vi "WMI Shutdown.vi"() -> ()   [LabVIEW 2012]
uses:
  System.Management
panel:
  out "error out":errorcluster
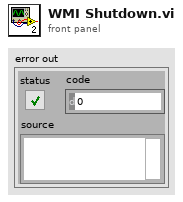
[diagram p1: front panel]
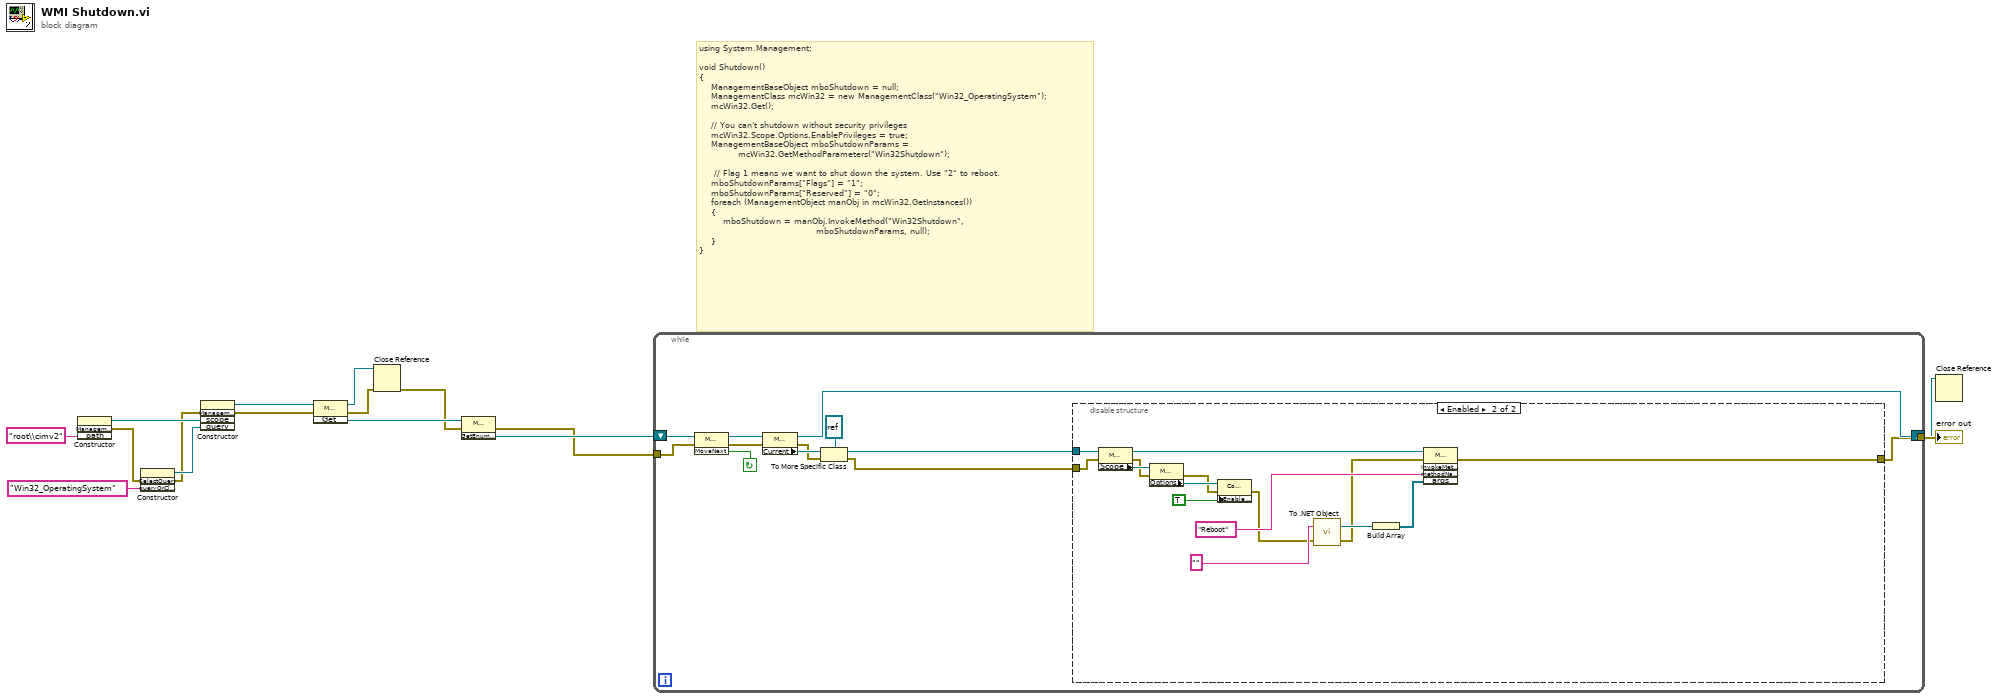
[diagram p0: block diagram]
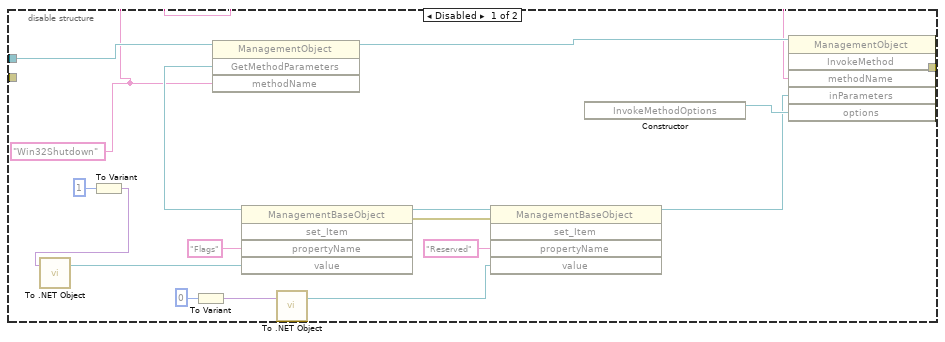
[diagram p2: hidden frame]
diagram:
  # "using System.Management;\n\nvoid Shutdown()\n{\n    ManagementBaseObject mboShutdown = null;\n    ManagementClass mcWin32 = new ManagementClass(\"Win32_OperatingSystem\");\n    mcWin32.Get();\n\n    // You can't shutdown without security privileges\n    mcWin32.Scope.Options.EnablePrivileges = true;\n    ManagementBaseObject mboShutdownParams =\n             mcWin32.GetMethodParameters(\"Win32Shutdown\");\n\n     // Flag 1 means we want to shut down the system. Use \"2\" to reboot.\n    mboShutdownParams[\"Flags\"] = \"1\";\n    mboShutdownParams[\"Reserved\"] = \"0\";\n    foreach (ManagementObject manObj in mcWin32.GetInstances())\n    {\n        mboShutdown = manObj.InvokeMethod(\"Win32Shutdown\", \n                                       mboShutdownParams, null);\n    }\n}"
  n1 = constructor class="ManagementScope"("path"="root\\cimv2" ("Scope")) -> (reference out=w14:refnum<k24>, error out=w2:errorcluster)  [unwired: 3 in, 2 out]
  n2 = constructor class="SelectQuery"(error in=w2, "queryOrClassName"="Win32_OperatingSystem") -> (reference out=w13:refnum<k24>, error out=w1:errorcluster)  [unwired: 2 in, 2 out]
  n3 = constructor class="ManagementObjectSearcher"(error in=w1, "scope"=w14, "query"=w13) -> (reference out=w3:refnum<k24>, error out=w10:errorcluster)  [unwired: 2 in, 3 out]
  n4 = invoke class="ManagementObjectSearcher" method="Get"(reference=w3, error in=w10) -> (reference out=w7:refnum<k24>, error out=w6:errorcluster, "Get"=w12:refnum<k24>)  [unwired: 1 in]
  n5 = Close Reference(reference=w7, error in (no error)=w6) -> (error out=w5:errorcluster)
  n6 = invoke class="ManagementObjectCollection" method="GetEnumerator"(reference=w12, error in=w5) -> (error out=w9:errorcluster, "GetEnumerator"=w11:refnum<k24>)  [unwired: 1 in, 1 out]
  n7 = while {
    shift-right: [w24] -> w4
    shift-left: w11 -> [w28]
    tunnel: w9 -> [w21]
    tunnel: [w18] -> w8
    stop <- w27 continue-if-true
    n8 = invoke class="ManagementObjectCollection+Mana" method="MoveNext"(reference=w28, error in=w21) -> (reference out=w25:refnum<k24>, error out=w20:errorcluster, "MoveNext"=w27:bool)  [unwired: 1 in]
    n9 = property class="ManagementObjectCollection+Mana"(reference=w25, error in=w20) -> (reference out=w24:refnum<k24>, error out=w22:errorcluster, "Current"=w23:refnum<k24>)
    n10 = To More Specific Class(target class=refnum<k24> refnum ("Current"), reference=w23, error in=w22) -> (specific class reference=w19:refnum<k24>, error out=w17:errorcluster)
    n11 = disable-structure shown="Enabled" {
      disable-tunnel: [w45 w56] -> w18
      disable-tunnel: w19 -> [w44 w55]
      disable-tunnel: w17 -> [_ w48]
      frame Disabled {
        w29 = "Win32Shutdown" ("propertyName")
        n12 = To Variant(anything=1) -> (Variant=w30:variant)
        n13 = call <vilib>:"To .NET Object.vi"("anything"=w30) -> (".NET object"=w41:refnum<k24>)  [unwired: 1 in, 1 out]
        n14 = To Variant(anything=0) -> (Variant=w37:variant)
        n15 = invoke class="ManagementObject" method="GetMethodParameters"(reference=w44, "methodName"=w29) -> (reference out=w34:refnum<k24>, "GetMethodParameters"=w43:refnum<k24>)  [unwired: 2 in, 2 out]
        n16 = invoke class="ManagementBaseObject" method="set_Item"(reference=w43, "propertyName"="Flags", "value"=w41) -> (reference out=w40:refnum<k24>, error out=w39:errorcluster)  [unwired: 2 in, 3 out]
        n17 = call <vilib>:"To .NET Object.vi"("anything"=w37) -> (".NET object"=w35:refnum<k24>)  [unwired: 1 in, 1 out]
        n18 = invoke class="ManagementBaseObject" method="set_Item"(reference=w40, error in=w39, "propertyName"="Reserved", "value"=w35) -> (reference out=w32:refnum<k24>)  [unwired: 1 in, 4 out]
        n19 = constructor class="InvokeMethodOptions"() -> (reference out=w33:refnum<k24>)  [unwired: 3 in, 2 out]
        n20 = invoke class="ManagementObject" method="InvokeMethod"(reference=w34, "methodName"=w29, "inParameters"=w32, "options"=w33) -> (error out=w45:errorcluster)  [unwired: 2 in, 5 out]
      }
      frame Enabled {
        n21 = property class="ManagementObject"(reference=w55, error in=w48) -> (reference out=w50:refnum<k24>, error out=w51:errorcluster, "Scope"=w54:refnum<k24>)
        n22 = property class="ManagementScope"(reference=w54, error in=w51) -> (error out=w49:errorcluster, "Options"=w53:refnum<k24>)  [unwired: 1 out]
        n23 = property class="ConnectionOptions"(reference=w53, error in=w49, "EnablePrivileges"=TRUE) -> (error out=w47:errorcluster)  [unwired: 1 out]
        n24 = call <vilib>:"To .NET Object.vi"("error in (no error)"=w47, "anything"="" ("methodName")) -> ("error out"=w46:errorcluster, ".NET object"=w58:refnum<k24>)
        n25 = Build Array(w58) -> (w57:refnum<k24>[])
        n26 = invoke class="ManagementObject" method="InvokeMethod"(reference=w50, error in=w46, "methodName"="Reboot", "args"=w57) -> (error out=w56:errorcluster)  [unwired: 1 in, 4 out]
      }
    }
  }
  "error out" <- w8
  n27 = Close Reference(reference=w4) -> ()  [unwired: 1 in, 1 out]
